vi "Output Waveform Configuration.vi"(0 "Refnum in":refnum<k20>, 1 "processing mode":T1, 5 "output stream instance":u32=1, 7 "waveform config":T2(array[cluster])=[{"Frequency (Hz)"=200000000.0, "Amplitude (V)"=0.4, "Phase (Deg)"=0.0}, {"Frequency (Hz)"=200000000.0, "Amplitude (V)"=0.4, "Phase (Deg)"=0.0}] {"Phase (Deg)" format="%.2p"; "Amplitude (V)" format="%0.2p"; "Frequency (Hz)" format="%0.2p"}, 11 "error in (no error)":errorcluster, 12 "DUC Frequency Shift":dbl) -> (4 "Refnum out":refnum<k20>, 6 "output stream instance out":u32=1, 8 "waveforms out":waveform(dbl)[](array[waveform]), 13 "ao wfm samples":i32, 15 "error out":errorcluster)   [LabVIEW 2018, in "GettingStarted_5785_Host.lvlib"]
uses:
  GettingStarted_5785_Host.lvlib
  Upconversion Mode.ctl
  <instrlib>/FlexRIO/API/Host/v1/NI FlexRIO/API/Get Property Reference - Fpga Small.vi
  <resource>/objmgr/niflexrioapiStream.rc
  <instrlib>/FlexRIO/API/Host/v1/NI FlexRIO API v1.lvlib
  <resource>/objmgr/niflexrioapiChannel.rc
  <vilib>/gmath/NI_Gmath.lvlib
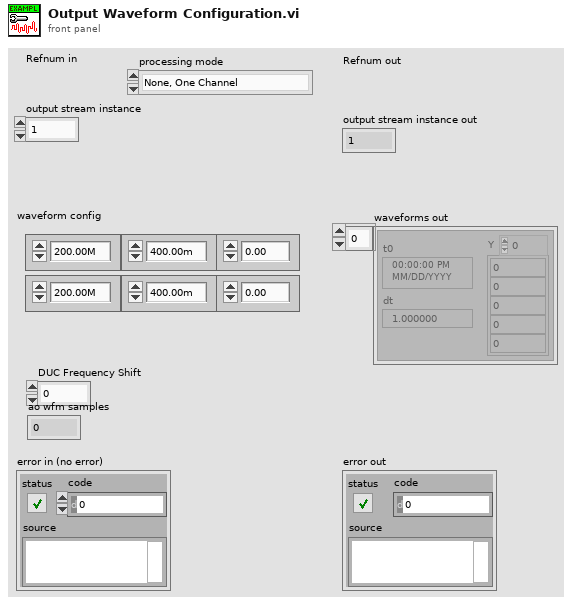
[diagram p1: front panel]
types:
  T1 = typedef "GettingStarted_5785_Host.lvlib/Upconversion Mode.ctl" = enum16{"None, One Channel", "None, Two Channels", "FPGA-only, One Channel", "DAC and FPGA, One Channel", "DAC-only, One Channel"}
  T2 = cluster{"Frequency (Hz)":dbl, "Amplitude (V)":dbl, "Phase (Deg)":dbl}[]
  T3 = cluster{"Frequency (Hz)":dbl, "Amplitude (V)":dbl, "Phase (Deg)":dbl}
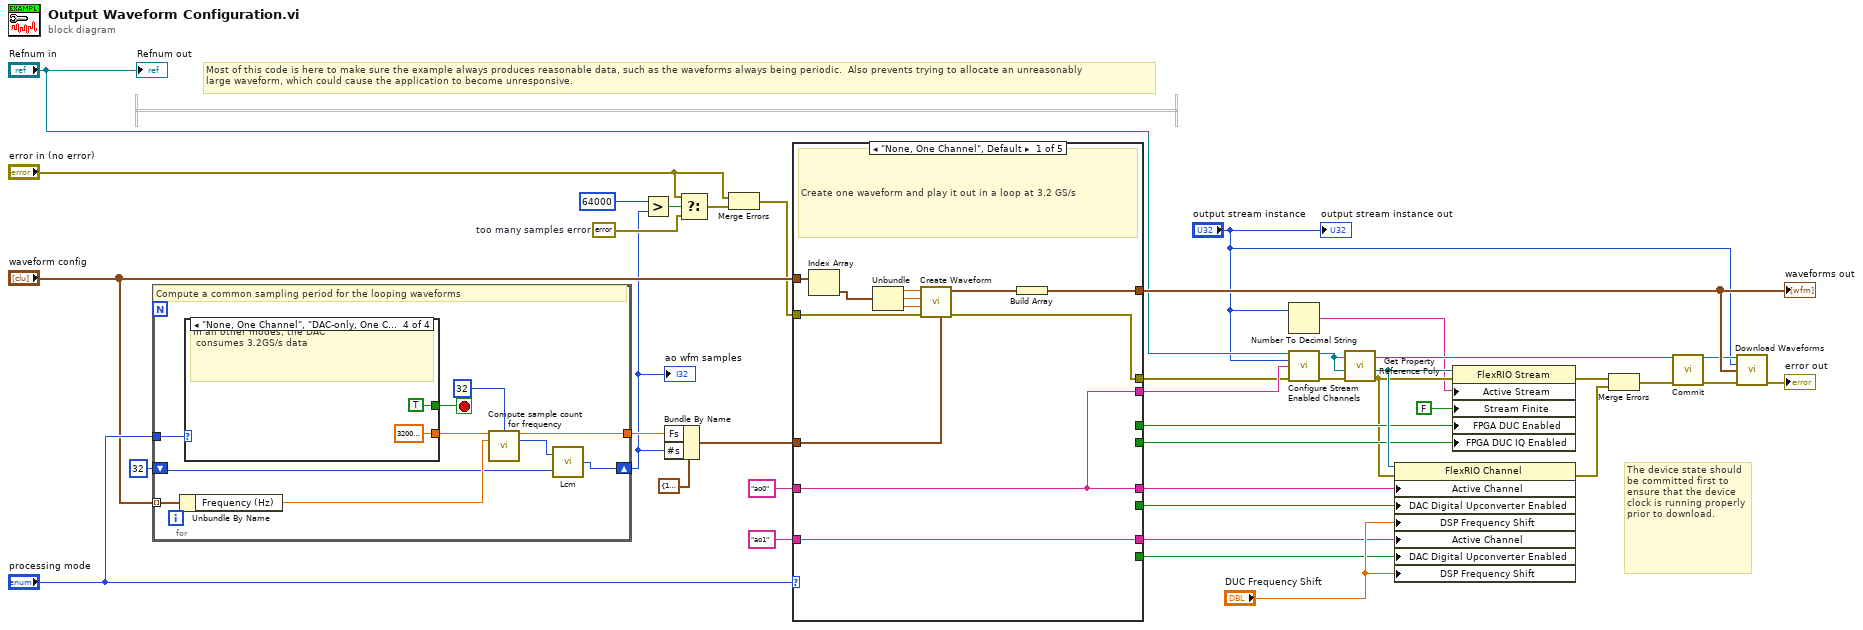
[diagram p0: block diagram]
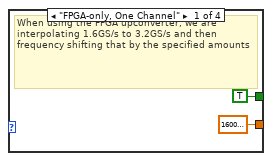
[diagram p2: hidden frame]
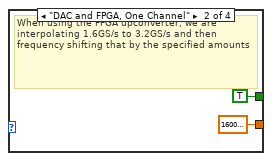
[diagram p3: hidden frame]
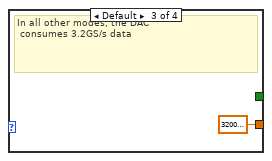
[diagram p4: hidden frame]
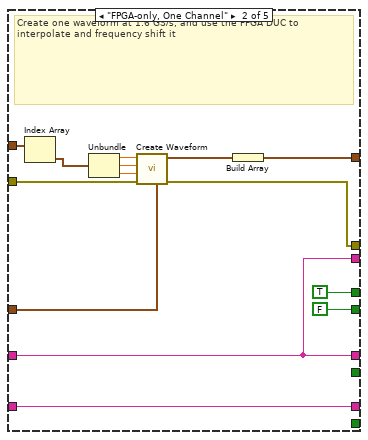
[diagram p5: hidden frame]
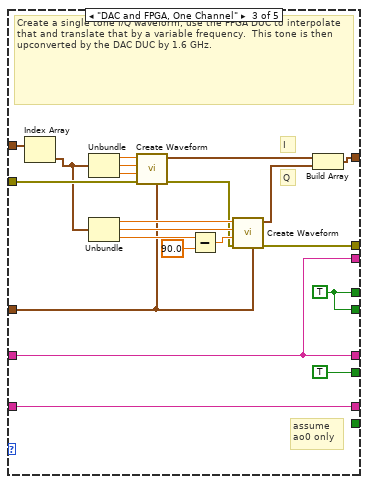
[diagram p6: hidden frame]
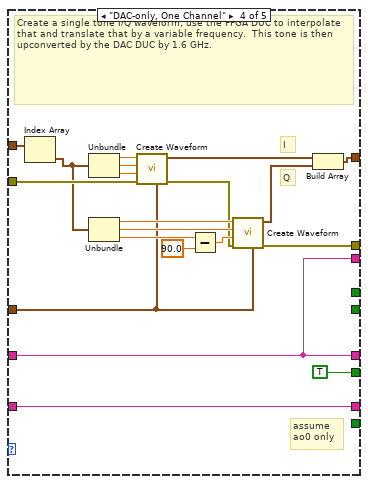
[diagram p7: hidden frame]
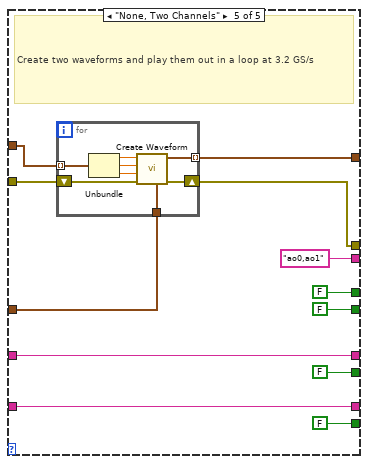
[diagram p8: hidden frame]
diagram:
  w5 = errorcluster {"status"=TRUE, "code"=0, "source"="Example code skipped waveform generation due to too many samples."}  # too many samples error
  # "Most of this code is here to make sure the example always produces reasonable data, such as the waveforms always being periodic.  Also prevents trying to allocate an unreasonably\nlarge waveform, which could cause the application to become unresponsive."
  # "The device state should be committed first to ensure that the device clock is running properly prior to download."
  n1 = for {
    tunnel: "processing mode" -> [w48]
    tunnel: "waveform config" -> [w47] mode=indexing
    shift-right: [w45] -> w1
    shift-left: i64 32 -> [w44]
    tunnel: [w40] -> w12
    stop <- w43 stop-if-true
    # "Compute a common sampling period for the looping waveforms"
    n2 = Unbundle By Name(w47) -> ("Frequency (Hz)"=w46:dbl)
    n3 = case shown="\"None, One Channel\", \"DAC-only, One Channel\"" w48 {
      tunnel: [1600000000.0 1600000000.0 3200000000.0 3200000000.0] -> w41
      tunnel: [TRUE TRUE _ TRUE] -> w43
      frame "FPGA-only, One Channel" {
        # "When using the FPGA upconverter, we are interpolating 1.6GS/s to 3.2GS/s and then frequency shifting that by the specified amounts"
      }
      frame "DAC and FPGA, One Channel" {
        # "When using the FPGA upconverter, we are interpolating 1.6GS/s to 3.2GS/s and then frequency shifting that by the specified amounts"
      }
      frame Default {
        # "In all other modes, the DAC\n consumes 3.2GS/s data"
      }
      frame "None, One Channel", "DAC-only, One Channel" {
        # "In all other modes, the DAC\n consumes 3.2GS/s data"
      }
    }
    n4 = call "Compute sample count for frequency.vi"("F (sampler)"=w41, "Sample Quantum"=32, "desired wfm frequency"=w46) -> ("F (sampler) out"=w40:dbl, "least common num samples"=w42:i64)  [unwired: 11 in]
    n5 = call <vilib>:"Lcm.vi"("y"=w44, "x"=w42) -> ("lcm(x,y)"=w45:i64)
  }
  "ao wfm samples" <- w1
  n6 = Greater?(x=i64 64000, y=w1) -> (0:w7:bool)
  n7 = Bundle By Name(cluster=cluster{"Fs":dbl, "#s":dbl} {"Fs"=100000000.0, "#s"=4000.0} ("sampling info"), "Fs"=w12, "#s"=w1) -> (w39:cluster{"Fs":dbl, "#s":dbl})
  n8 = Select(t="error in (no error)", s=w7, f=w5) -> (s? t:f=w6:errorcluster)
  n9 = Merge Errors("error in (no error)", w6) -> (w8:errorcluster)
  n10 = case shown="\"None, One Channel\", Default" "processing mode" {
    tunnel: "waveform config" -> [w68 w82 w103 w123 w135]
    tunnel: w8 -> [w63 w77 w99 w119 w133]
    tunnel: [w61 w75 w97 w117 w134] -> w24
    tunnel: "ao0" ("AO channel") -> [w60 w74 w96 w116 w129]
    tunnel: [w60 w74 w96 w116 "ao0,ao1" ("AO channel")] -> w26
    tunnel: "ao1" ("AO channel") -> [w59 w73 w95 w115 w128]
    tunnel: [_ TRUE w86 _ FALSE] -> w28
    tunnel: [_ FALSE w86 _ FALSE] -> w29
    tunnel: [w60 w74 w96 w116 w129] -> w31
    tunnel: [w59 w73 w95 w115 w128] -> w32
    tunnel: [_ _ TRUE ("Analog Output:DAC Digital Upconverter Enabled") TRUE ("Analog Output:DAC Digital Upconverter Enabled") FALSE ("Analog Output:DAC Digital Upconverter Enabled")] -> w33
    tunnel: [_ _ _ _ FALSE ("Analog Output:DAC Digital Upconverter Enabled")] -> w34
    tunnel: w39 -> [w58 w72 w84 w105 w125]
    tunnel: [w57 w70 w83 w104 w124] -> w18
    frame "None, One Channel", Default {
      # "Create one waveform and play it out in a loop at 3.2 GS/s"
      n11 = Index Array(array=w68) -> (element=w67:T3)  [unwired: 1 in]
      n12 = Unbundle(w67) -> ("Frequency (Hz)"=w66:dbl, "Amplitude (V)"=w65:dbl, "Phase (Deg)"=w64:dbl)
      n13 = call "Create Waveform.vi"("sampling info"=w58, "error in (no error)"=w63, "phase"=w64, "amplitude"=w65, "frequency"=w66) -> ("error out"=w57:errorcluster, "Output Waveform (V)"=w62:waveform(dbl))  [unwired: 4 in, 1 out]
      n14 = Build Array(w62) -> (w61:waveform(dbl)[])
    }
    frame "FPGA-only, One Channel" {
      # "Create one waveform at 1.6 GS/s, and use the FPGA DUC to interpolate and frequency shift it"
      n15 = Index Array(array=w82) -> (element=w81:T3)  [unwired: 1 in]
      n16 = Unbundle(w81) -> ("Frequency (Hz)"=w80:dbl, "Amplitude (V)"=w79:dbl, "Phase (Deg)"=w78:dbl)
      n17 = call "Create Waveform.vi"("sampling info"=w72, "error in (no error)"=w77, "phase"=w78, "amplitude"=w79, "frequency"=w80) -> ("error out"=w70:errorcluster, "Output Waveform (V)"=w76:waveform(dbl))  [unwired: 4 in, 1 out]
      n18 = Build Array(w76) -> (w75:waveform(dbl)[])
    }
    frame "DAC and FPGA, One Channel" {
      w86 = TRUE
      # "assume\nao0 only"
      # "Q"
      # "I"
      # "Create a single tone I/Q waveform, use the FPGA DUC to interpolate that and translate that by a variable frequency.  This tone is then upconverted by the DAC DUC by 1.6 GHz."
      n19 = Index Array(array=w103) -> (element=w93:T3)  [unwired: 1 in]
      n20 = Unbundle(w93) -> ("Frequency (Hz)"=w102:dbl, "Amplitude (V)"=w101:dbl, "Phase (Deg)"=w100:dbl)
      n21 = Unbundle(w93) -> ("Frequency (Hz)"=w94:dbl, "Amplitude (V)"=w92:dbl, "Phase (Deg)"=w91:dbl)
      n22 = call "Create Waveform.vi"("sampling info"=w84, "error in (no error)"=w99, "phase"=w100, "amplitude"=w101, "frequency"=w102) -> ("error out"=w87:errorcluster, "Output Waveform (V)"=w98:waveform(dbl))  [unwired: 4 in, 1 out]
      n23 = Subtract(x=w91, y=90.0) -> (x-y=w90:dbl)
      n24 = call "Create Waveform.vi"("sampling info"=w84, "error in (no error)"=w87, "phase"=w90, "amplitude"=w92, "frequency"=w94) -> ("error out"=w83:errorcluster, "Output Waveform (V)"=w88:waveform(dbl))  [unwired: 4 in, 1 out]
      n25 = Build Array(w98, w88) -> (w97:waveform(dbl)[])
    }
    frame "DAC-only, One Channel" {
      # "assume\nao0 only"
      # "Q"
      # "I"
      # "Create a single tone I/Q waveform, use the FPGA DUC to interpolate that and translate that by a variable frequency.  This tone is then upconverted by the DAC DUC by 1.6 GHz."
      n26 = Index Array(array=w123) -> (element=w113:T3)  [unwired: 1 in]
      n27 = Unbundle(w113) -> ("Frequency (Hz)"=w122:dbl, "Amplitude (V)"=w121:dbl, "Phase (Deg)"=w120:dbl)
      n28 = Unbundle(w113) -> ("Frequency (Hz)"=w114:dbl, "Amplitude (V)"=w112:dbl, "Phase (Deg)"=w111:dbl)
      n29 = call "Create Waveform.vi"("sampling info"=w105, "error in (no error)"=w119, "phase"=w120, "amplitude"=w121, "frequency"=w122) -> ("error out"=w107:errorcluster, "Output Waveform (V)"=w118:waveform(dbl))  [unwired: 4 in, 1 out]
      n30 = Subtract(x=w111, y=90.0) -> (x-y=w110:dbl)
      n31 = call "Create Waveform.vi"("sampling info"=w105, "error in (no error)"=w107, "phase"=w110, "amplitude"=w112, "frequency"=w114) -> ("error out"=w104:errorcluster, "Output Waveform (V)"=w108:waveform(dbl))  [unwired: 4 in, 1 out]
      n32 = Build Array(w118, w108) -> (w117:waveform(dbl)[])
    }
    frame "None, Two Channels" {
      # "Create two waveforms and play them out in a loop at 3.2 GS/s"
      n33 = for {
        tunnel: w135 -> [w140] mode=indexing
        tunnel: [w139] -> w134 mode=indexing
        shift-right: [w137] -> w124
        shift-left: w133 -> [w138]
        tunnel: w125 -> [w136]
        n34 = Unbundle(w140) -> ("Frequency (Hz)"=w143:dbl, "Amplitude (V)"=w142:dbl, "Phase (Deg)"=w141:dbl)
        n35 = call "Create Waveform.vi"("sampling info"=w136, "error in (no error)"=w138, "phase"=w141, "amplitude"=w142, "frequency"=w143) -> ("error out"=w137:errorcluster, "Output Waveform (V)"=w139:waveform(dbl))  [unwired: 4 in, 1 out]
      }
    }
  }
  "waveforms out" <- w24
  n36 = Number To Decimal String(number="output stream instance") -> (decimal integer string=w3:string)  [unwired: 1 in]
  n37 = call <instrlib>:"Configure Stream Enabled Channels.vi"("fpga interface in"="Refnum in", "stream instance"="output stream instance", "channels enabled"=w26, "error in"=w18) -> ("fpga interface out"=w19:refnum<k20>, "error out"=w22:errorcluster)  [unwired: 8 in, 2 out]
  n38 = call-poly <instrlib>:"Get Property Reference Poly.vi"("error in (no error)"=w22, "fpga interface in"=w19) -> ("error out"=w21:errorcluster, "property reference"=w30:refnum<k20>)  [unwired: 4 in, 1 out]
  n39 = property class="FlexRIO Channel"(reference=w30, error in=w21, "Active Channel"=w31, "DAC Digital Upconverter Enabled"=w33, "DSP Frequency Shift"="DUC Frequency Shift", "Active Channel"=w32, "DAC Digital Upconverter Enabled"=w34, "DSP Frequency Shift"="DUC Frequency Shift") -> (error out=w36:errorcluster)  [unwired: 1 out]
  n40 = property class="FlexRIO Stream"(reference=w30, error in=w21, "Active Stream"=w3, "Stream Finite"=FALSE ("Configuration:Finite"), "FPGA DUC Enabled"=w28, "FPGA DUC IQ Enabled"=w29) -> (error out=w37:errorcluster)  [unwired: 1 out]
  n41 = Merge Errors(w37, w36) -> (w20:errorcluster)
  n42 = call <instrlib>:"Commit.vi"("fpga interface in"=w19, "error in"=w20) -> ("fpga interface out"=w17:refnum<k20>, "error out"=w16:errorcluster)  [unwired: 12 in]
  n43 = call "Download Waveforms.vi"("fpga interface in"=w17, "stream instance"="output stream instance", "waveforms"=w24, "error in"=w16) -> ("error out"=→"error out":errorcluster)  [unwired: 9 in, 2 out]
  "Refnum out" <- "Refnum in"
  "output stream instance out" <- "output stream instance"
